vi "Base64 to String2.vi"(6 "error in (no error)":errorcluster, 10 "Base64 String":string) -> (2 "String":string, 4 "error out":errorcluster)   [LabVIEW 2016, in "数据传输系统.lvlib"]
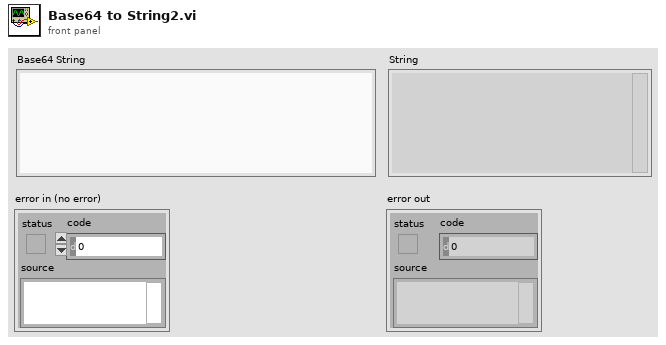
[diagram p1: front panel]
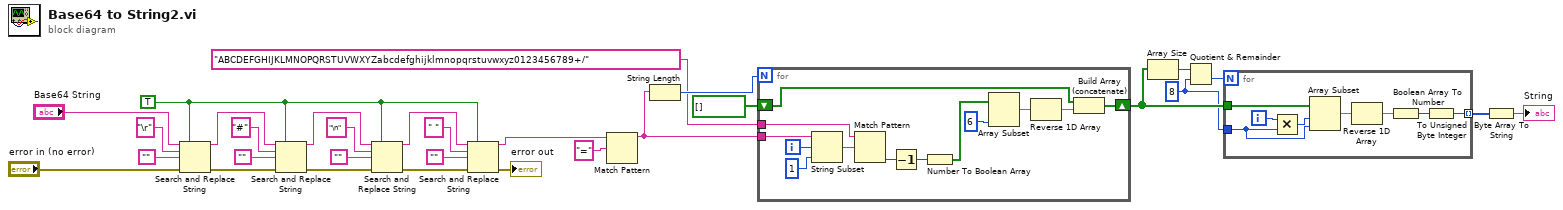
[diagram p0: block diagram]
diagram:
  w4 = TRUE ("replace all? (F)")
  w22 = 8 ("y")
  n1 = Search and Replace String(replace all?=w4, input string="Base64 String", search string="\r" ("replace string (\"\")"), replace string="", error in="error in (no error)") -> (result string=w5:string, error out=w3:errorcluster)  [unwired: 5 out]
  n2 = Search and Replace String(replace all?=w4, input string=w5, search string="#" ("replace string (\"\")"), replace string="", error in=w3) -> (result string=w1:string, error out=w2:errorcluster)  [unwired: 5 out]
  n3 = Search and Replace String(replace all?=w4, input string=w1, search string="\n" ("replace string (\"\")"), replace string="", error in=w2) -> (result string=w11:string, error out=w10:errorcluster)  [unwired: 5 out]
  n4 = Search and Replace String(replace all?=w4, input string=w11, search string=" " ("replace string (\"\")"), replace string="", error in=w10) -> (result string=w8:string, error out=→"error out":errorcluster)  [unwired: 5 out]
  n5 = Match Pattern(string=w8, regular expression="=") -> (before substring=w27:string)  [unwired: 4 out]
  n6 = String Length(string=w27) -> (length=w30:i32)
  n7 = for {
    N: w30 -> [_]
    tunnel: w27 -> [w43]
    tunnel: "ABCDEFGHIJKLMNOPQRSTUVWXYZabcdefghijklmnopqrstuvwxyz0123456789+/" -> [w40]
    shift-right: [w33] -> w23
    shift-left: bool[] [] -> [w32]
    i -> [w41]
    n8 = String Subset(string=w43, offset (0)=w41, length (rest)=1 ("length (rest)")) -> (substring=w39:string)
    n9 = Match Pattern(string=w40, regular expression=w39) -> (offset past match=w38:i32)  [unwired: 1 in, 3 out]
    n10 = Decrement(x=w38) -> (x-1=w37:i32)
    n11 = Number To Boolean Array(number=w37) -> (Boolean array=w36:bool[])
    n12 = Array Subset(array=w36, length=6) -> (w34:bool[])  [unwired: 1 in]
    n13 = Reverse 1D Array(array=w34) -> (reversed array=w31:bool[])
    n14 = Build Array (concatenate)(w32, w31) -> (w33:bool[])
  }
  n15 = Array Size(array=w23) -> (size(s)=w25:i32)
  n16 = Quotient & Remainder(x=w25, y=w22) -> (floor(x/y)=w24:i32)  [unwired: 1 out]
  n17 = for {
    N: w24 -> [_]
    tunnel: w23 -> [w51]
    tunnel: w22 -> [w50]
    tunnel: [w46] -> w21 mode=indexing
    i -> [w49]
    n18 = Multiply(x=w49, y=w50) -> (x*y=w44:i32)
    n19 = Array Subset(array=w51, index=w44, length=w50) -> (w48:bool[])
    n20 = Reverse 1D Array(array=w48) -> (reversed array=w45:bool[])
    n21 = Boolean Array To Number(Boolean array=w45) -> (number=w47:u32)
    n22 = To Unsigned Byte Integer(number=w47) -> (unsigned 8bit integer=w46:u8)
  }
  n23 = Byte Array To String(unsigned byte array=w21) -> (string=→"String":string)
